vi "niDTS WLAN INSTR TX Configure TXP.vi"(8 "error in (no error)":errorcluster, 11 "niDTS WLAN INSTR TX in":refnum<class "niDTS WLAN INSTR TX.lvclass">) -> (0 "error out":errorcluster, 3 "niDTS WLAN INSTR TX out":refnum<class "niDTS WLAN INSTR TX.lvclass">)   [LabVIEW 2015, in "niDTS WLAN.lvlib" / "niDTS WLAN INSTR TX.lvclass"]
doc: "Sets:\n\n* TxPowerEnabled\n* NumberOfAverages(txp)\n* MeasurementMode"
uses:
  niDTS WLAN INSTR TX.lvclass
  niDTS WLAN INSTR TX.lvclass/niDTS WLAN INSTR TX.ctl
  RiviInstDriver/niRfsaWlan/Objects/niRfsaWlan.lvclass
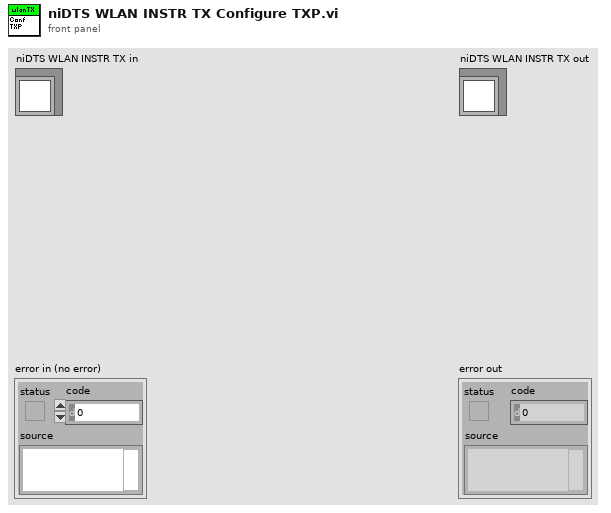
[diagram p1: front panel]
types:
  T1 = typedef "niRfsaWlan.lvclass/niRfsaWlan INC Handle.ctl" = refnum<data-value>
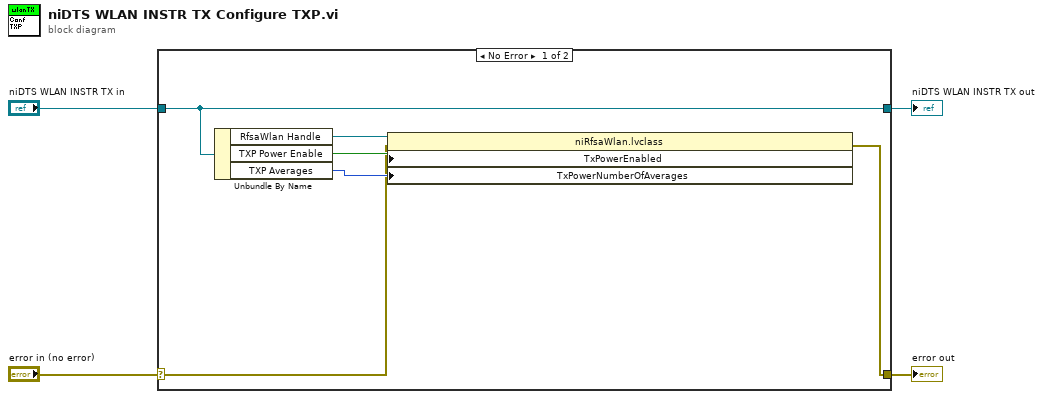
[diagram p0: block diagram]
diagram:
  n1 = case shown="No Error" "error in (no error)" {
    selector: "error in (no error)" -> [w6 w12]
    tunnel: [w5 w12] -> w3
    tunnel: [w10 w11] -> w1
    tunnel: "niDTS WLAN INSTR TX in" -> [w10 w11]
    frame No Error {
      n2 = Unbundle By Name(w10) -> ("RfsaWlan Handle"=w9:T1, "TXP Power Enable"=w8:bool, "TXP Averages"=w7:i32)
      n3 = property class="niRfsaWlan.lvclass"(reference=w9, error in=w6, "TxPowerEnabled"=w8, "TxPowerNumberOfAverages"=w7) -> (error out=w5:errorcluster)  [unwired: 1 out]
    }
    frame Error {
    }
  }
  "error out" <- w3
  "niDTS WLAN INSTR TX out" <- w1
